vi "RedistributeArmPathPointsVariable.vi"(1 "DesiredPointSpacing":dbl[](array[numeric]), 2 "ArmPathIn":T1[](array[typedef]), 3 "IndexedPathLength":dbl[](array[numeric])) -> (0 "ArmPathOut":T1[](array[typedef]))   [LabVIEW 2017]
uses:
  TypeDefs/ArmCoordinate.ctl
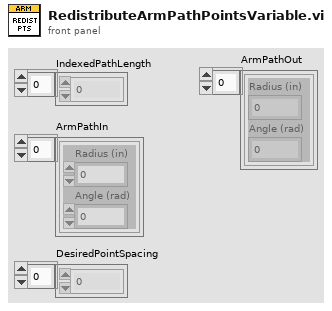
[diagram p1: front panel]
types:
  T1 = typedef "ArmCoordinate.ctl" = cluster{"Radius (in)":dbl, "Angle (rad)":dbl}
  T2 = typedef "Point2D.ctl" = cluster{"X":dbl, "Y":dbl}
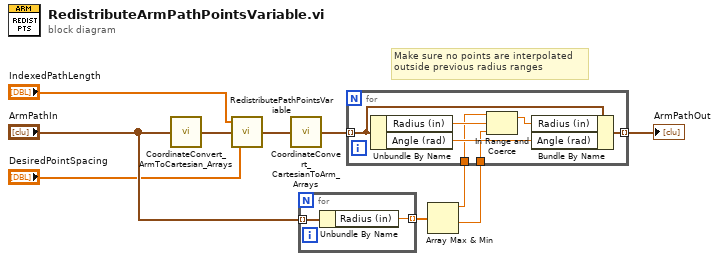
[diagram p0: block diagram]
diagram:
  # "Make sure no points are interpolated\noutside previous radius ranges"
  n1 = call "CoordinateConvert_ArmToCartesian_Arrays.vi"("ArmCoordinates"="ArmPathIn") -> ("XYPoints"=w3:T2[])
  n2 = call "RedistributePathPointsVariable.vi"("DesiredPointSpacing"="DesiredPointSpacing", "PathIn"=w3, "IndexedPathLength"="IndexedPathLength") -> ("PathOut"=w4:T2[])
  n3 = call "CoordinateConvert_CartesianToArm_Arrays.vi"("XYPoints"=w4) -> ("ArmCoordinates"=w8:T1[])
  n4 = for {
    tunnel: "ArmPathIn" -> [w12] mode=indexing
    tunnel: [w11] -> w10 mode=indexing
    n5 = Unbundle By Name(w12) -> ("Radius (in)"=w11:dbl)
  }
  n6 = Array Max & Min(array=w10) -> (max value=w6:dbl, min value=w5:dbl)  [unwired: 2 out]
  n7 = for {
    tunnel: w8 -> [w18] mode=indexing
    tunnel: [w19] -> w7 mode=indexing
    tunnel: w6 -> [w14]
    tunnel: w5 -> [w13]
    n8 = Unbundle By Name(w18) -> ("Radius (in)"=w15:dbl, "Angle (rad)"=w17:dbl)
    n9 = In Range and Coerce(upper limit=w14, x=w15, lower limit=w13) -> (coerced(x)=w16:dbl)  [unwired: 1 out]
    n10 = Bundle By Name(cluster=w18, "Radius (in)"=w16, "Angle (rad)"=w17) -> (w19:T1)
  }
  "ArmPathOut" <- w7
